vi "Create Python Graph.vi"(0 "File Name":string, 1 "Title":string, 2 "Main Side":bool, 3 "Wet Test":bool, 4 "Y-Axis Max":i32, 5 "LS Series":string, 7 "Error IN":errorcluster, 9 "Data Base Path":path, 12 "Init (F)":bool, 13 "Tolerances Path":path, 14 "X-Axis Min":i32, 15 "Python Script Directory":path=path "C:/Users/gtetil/Documents/Projects/ls-tester-graph-script", 16 "X-Axis Max (Height)":i32, 17 "Data Start Index":u32, 18 "X-Axis Max (Time)":i32) -> (20 "Command Line Error":string, 27 "Error OUT":errorcluster)   [LabVIEW 2013]
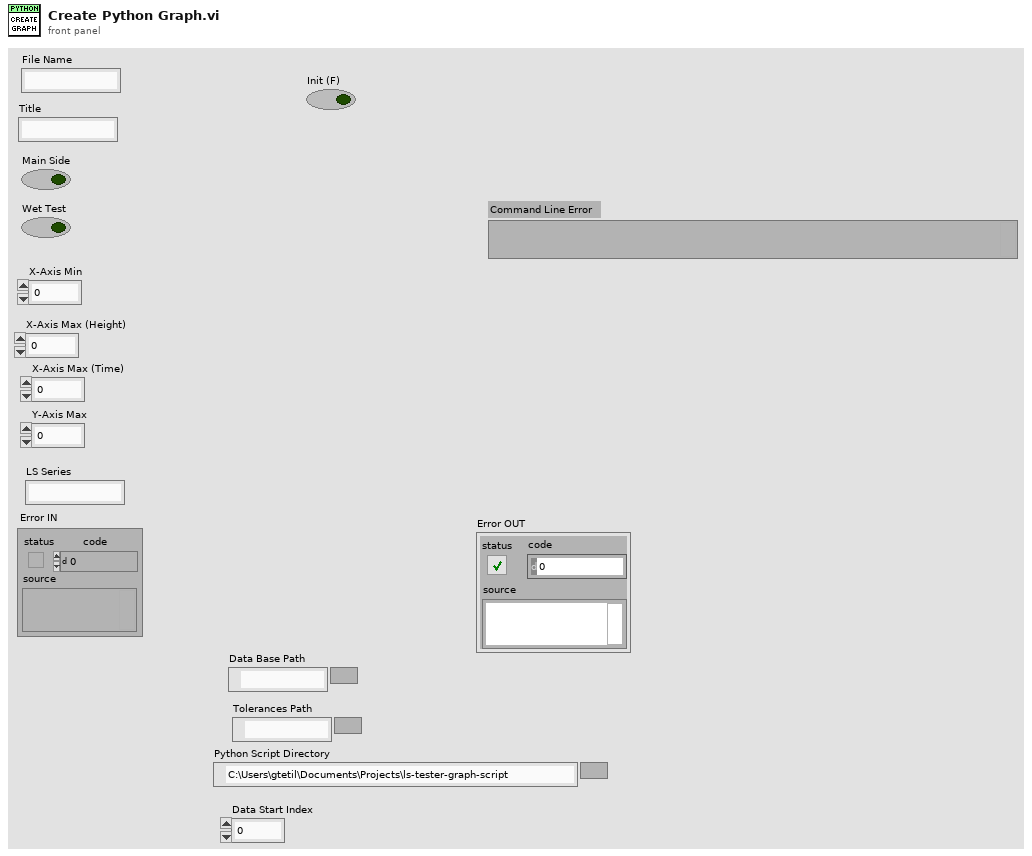
[diagram p1: front panel]
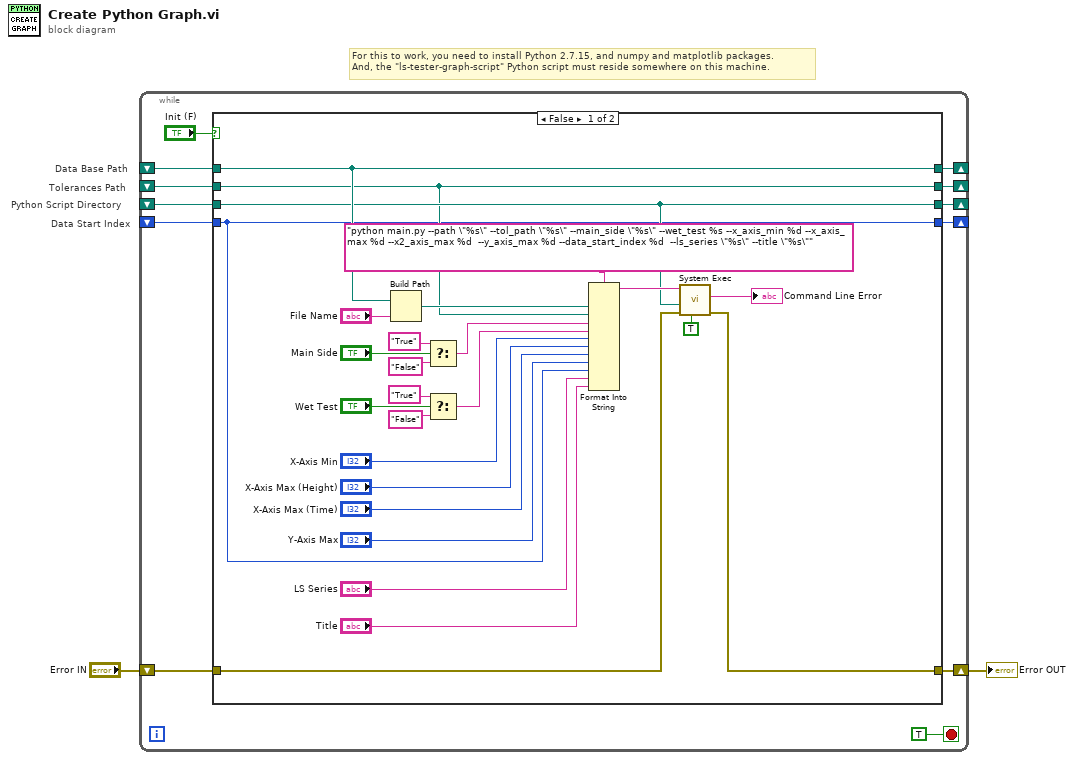
[diagram p0: block diagram]
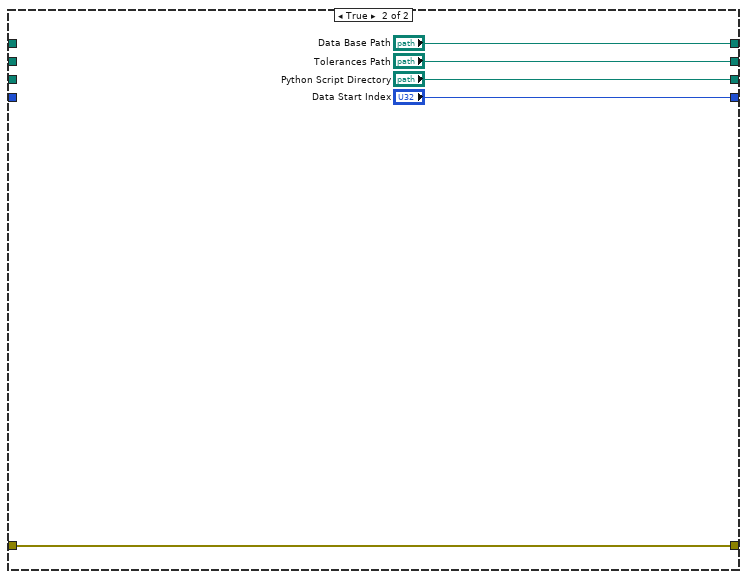
[diagram p2: hidden frame]
diagram:
  # "Tolerances Path"
  # "For this to work, you need to install Python 2.7.15, and numpy and matplotlib packages.\nAnd, the \"ls-tester-graph-script\" Python script must reside somewhere on this machine."
  # "Data Start Index"
  # "Python Script Directory"
  # "Data Base Path"
  n1 = while {
    shift-right: [w12] -> _
    shift-left: _ -> [w9]
    shift-right: [w11] -> _
    shift-left: _ -> [w8]
    shift-right: [w10] -> _
    shift-left: _ -> [w7]
    shift-right: [w5] -> w1
    shift-left: "Error IN" -> [w6]
    shift-right: [w4] -> _
    shift-left: _ -> [w3]
    stop <- TRUE stop-if-true
    n2 = case shown="False" "Init (F)" {
      tunnel: [w33 "Data Base Path"] -> w12
      tunnel: [w32 "Python Script Directory"] -> w11
      tunnel: [w20 "Data Start Index"] -> w10
      tunnel: w9 -> [w33 _]
      tunnel: w8 -> [w32 _]
      tunnel: w7 -> [w20 _]
      tunnel: w6 -> [w31 w42]
      tunnel: [w30 w42] -> w5
      tunnel: [w27 "Tolerances Path"] -> w4
      tunnel: w3 -> [w27 _]
      frame False {
        n3 = Build Path(base path=w33, name or relative path="File Name") -> (appended path=w34:path)
        n4 = Select(t="True", s="Main Side", f="False") -> (s? t:f=w22:string)
        n5 = Select(t="True", s="Wet Test", f="False") -> (s? t:f=w26:string)
        n6 = Format Into String(format string="python main.py --path \"%s\" --tol_path \"%s\" --main_side \"%s\" --wet_test %s --x_axis_min %d --x_axis_max %d --x2_axis_max %d  --y_axis_max %d --data_start_index %d  --ls_series \"%s\" --title \"%s\"", w34, w27, w22, w26, "X-Axis Min", "X-Axis Max (Height)", "X-Axis Max (Time)", "Y-Axis Max", w20, "LS Series", "Title") -> (resulting string=w39:string)  [unwired: 2 in, 1 out]
        n7 = call <vilib>:"System Exec.vi"("run minimized? (F)"=TRUE, "error in (no error)"=w31, "working directory"=w32, "command line"=w39) -> ("error out"=w30:errorcluster, "standard error"=→"Command Line Error":string)  [unwired: 4 in, 2 out]
      }
      frame True {
      }
    }
  }
  "Error OUT" <- w1
